vi "CTR_StartOutputFreq.vi"(7 "DeviceIndex":u32, 8 "error in (no error)":errorcluster, 10 "Output Frequency (Hz)":dbl, 11 "BlockIndex":u32) -> (0 "error out":errorcluster, 2 "Actual Frequency (Hz)":dbl)   [LabVIEW 2012]
doc: "unsigned long CTR_StartOutputFreq(\nunsigned long DeviceIndex - number from 0-31 indicating on which device you wish to output a\nfrequency\nunsigned long BlockIndex - number indicating which 8254 you wish to output a frequency from\ndouble *pHz - pointer to a double precision IEEE floating point number containing the desired\noutput frequency. This value is set by the driver to the actual frequency that will be output, as\nlimited by the device’s capabilities.\n)"
uses:
  Windows/System32/AIOUSB.dll
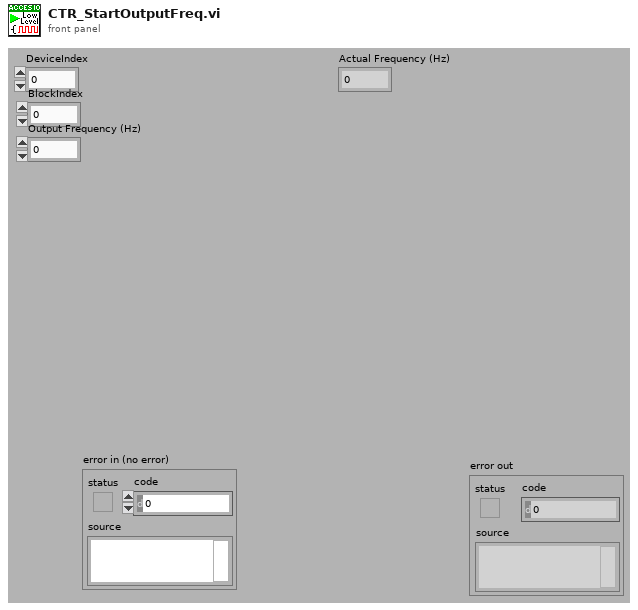
[diagram p1: front panel]
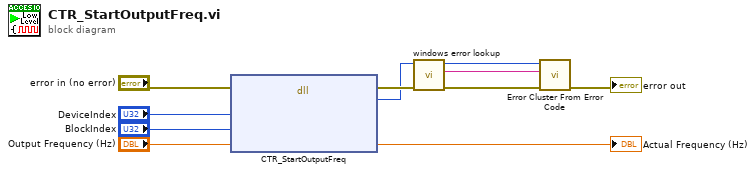
[diagram p0: block diagram]
diagram:
  n1 = dll-call lib="C:/Windows/System32/AIOUSB.dll" fn="CTR_StartOutputFreq"(error in="error in (no error)", "DeviceIndex"="DeviceIndex", "BlockIndex"="BlockIndex", "pHz"="Output Frequency (Hz)") -> (error out=w7:errorcluster, "return type"=w6:u32, "pHz"=→"Actual Frequency (Hz)":dbl)  [unwired: 4 in, 1 out]
  n2 = call "windows error lookup.vi"("error in (no error)"=w7, "Error Code"=w6) -> ("error out"=w9:errorcluster, "error message (\"\")"=w10:string)  [unwired: 8 in]
  n3 = call <vilib>:"Error Cluster From Error Code.vi"("error in (no error)"=w9, "error message (\"\")"=w10, "error code (0)"=w6) -> ("error out"=→"error out":errorcluster)  [unwired: 6 in]
